vi "RFID_TagEventExe.vi"(0 "Devices In":u64[](array[numeric]), 5 "Event Registration Refnum In":refnum<event-registration>, 11 "error in (no error)":errorcluster) -> (2 "Index":i32, 3 "Event?":bool, 4 "Devices Out":u64[](array[numeric]), 6 "Event Registration Refnum Out":refnum<event-registration>, 8 "Tag String":string, 10 "Protocol":i32(ring) items=["PROTOCOL_EM4100"=1, "PROTOCOL_ISO11785_FDX_B"=2, "PROTOCOL_PHIDGETS"=3], 14 "phid":u64, 15 "error out":errorcluster)   [LabVIEW 2012, in "Phidget RFID.lvlib"]
doc: "${Tag:Header}"
uses:
  <instrlib>/Phidgets/Phidget RFID/Phidget RFID.lvlib
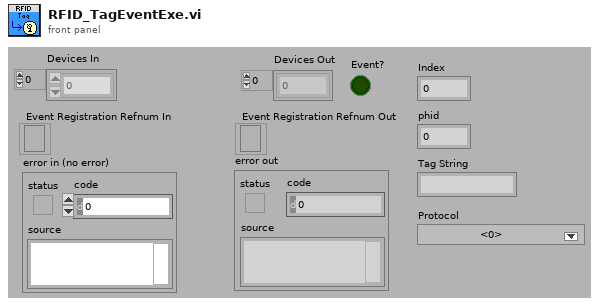
[diagram p1: front panel]
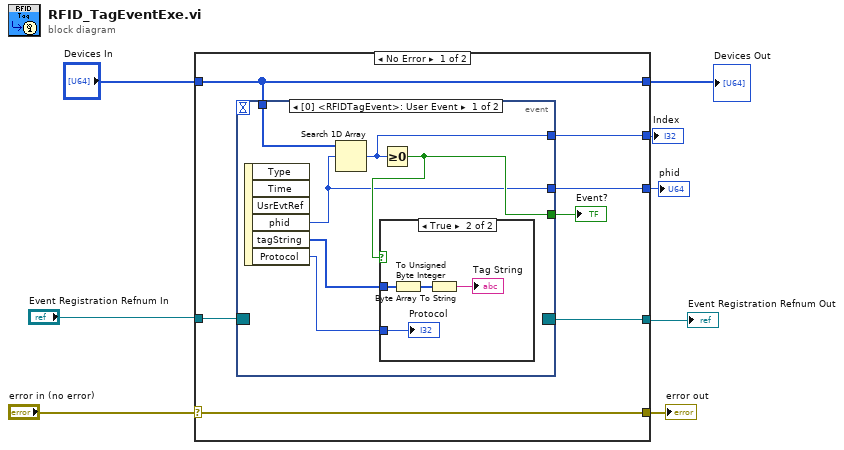
[diagram p0: block diagram]
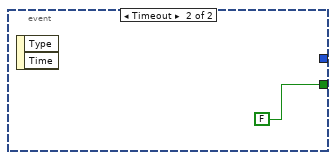
[diagram p3: hidden frame]
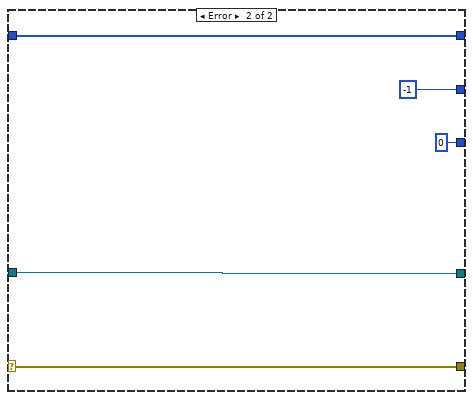
[diagram p4: hidden frame]
diagram:
  n1 = case shown="No Error" "error in (no error)" {
    selector: "error in (no error)" -> [w12 w31]
    tunnel: [w12 w31] -> w7
    tunnel: [w15 w30] -> w1
    tunnel: "Event Registration Refnum In" -> [w14 w30]
    tunnel: [w11 w29] -> w5
    tunnel: "Devices In" -> [w11 w29]
    tunnel: [w10 -1] -> w4
    tunnel: [w9 u64 0 ("phid")] -> w3
    frame No Error {
      n2 = event shown="[0] <RFIDTagEvent>: User Event" {
        selector: w14 -> [_ _]
        dyn-events: [_ _] -> w15
        timeout: _ -> [_ _]
        tunnel: [w20 FALSE] -> w13
        tunnel: w11 -> [w21 _]
        tunnel: [w19 _] -> w10
        tunnel: [w17 _] -> w9
        event User Event {
          n3 = event-data() -> ("phid"=w17:u64, "tagString"=w18:i8[], "Protocol"=w16:i32)  [unwired: 1 in, 3 out]
          n4 = Search 1D Array(1D array=w21, element=w17) -> (index of element=w19:i32)  [unwired: 1 in]
          n5 = Greater Or Equal To 0?(x=w19) -> (x >= 0?=w20:bool)
          n6 = case shown="True" w20 {
            tunnel: w18 -> [_ w23]
            tunnel: w16 -> [_ w25]
            frame False {
            }
            frame True {
              n7 = To Unsigned Byte Integer(number=w23) -> (unsigned 8bit integer=w22:u8[])
              n8 = Byte Array To String(unsigned byte array=w22) -> (string=→"Tag String":string)
              "Protocol" <- w25
            }
          }
        }
        event Timeout {
          n9 = event-data() -> ()  [unwired: 1 in, 2 out]
        }
      }
      "Event?" <- w13
    }
    frame Error {
    }
  }
  "error out" <- w7
  "Devices Out" <- w5
  "Index" <- w4
  "phid" <- w3
  "Event Registration Refnum Out" <- w1
